vi "get_double_check_moving_by_name.vi"(8 "error in (no error)":errorcluster, 10 "name":string, 11 "MotorSystem in":refnum<class "MotorSystem.lvclass">) -> (0 "error out":errorcluster, 2 "?":cluster{"1st check":bool, "2nd check":bool}, 3 "MotorSystem out":refnum<class "MotorSystem.lvclass">)   [LabVIEW 2016, in "MotionControl.lvlib" / "MotorSystem.lvclass"]
uses:
  <userlib>/MotionControl/MotorSystem/MotorSystem.lvclass
  <userlib>/MotionControl/MotorSystem/MotorSystem.lvclass/MotorSystem.ctl
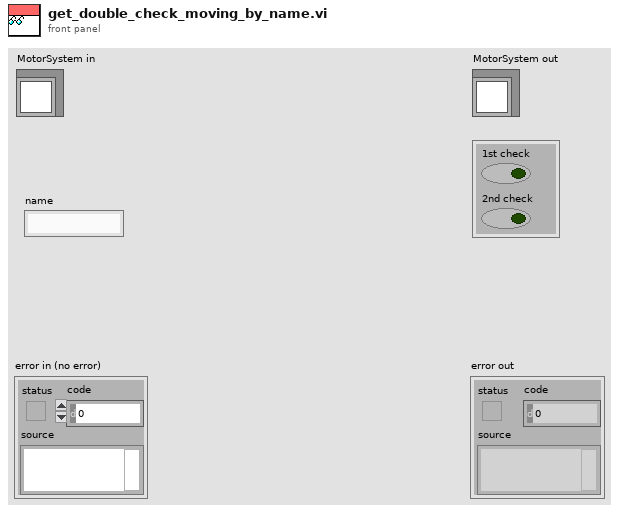
[diagram p1: front panel]
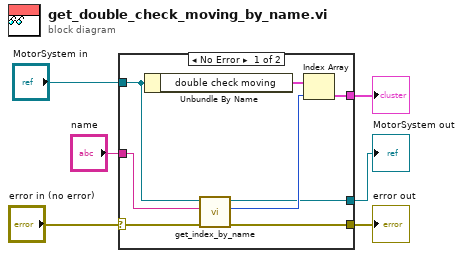
[diagram p0: block diagram]
diagram:
  n1 = case shown="No Error" "error in (no error)" {
    selector: "error in (no error)" -> [w9 w15]
    tunnel: [w8 w15] -> w5
    tunnel: [w7 w16] -> w3
    tunnel: "MotorSystem in" -> [w12 w16]
    tunnel: [w13 _] -> w2
    tunnel: "name" -> [w11 _]
    frame No Error {
      n2 = Unbundle By Name(w12) -> ("double check moving"=w14:cluster{"1st check":bool, "2nd check":bool}[])
      n3 = call <userlib>:"get_index_by_name.vi"("error in (no error)"=w9, "name"=w11, "MotorSystem 输入"=w12) -> ("error out"=w8:errorcluster, "index (0-based)"=w10:u32, "MotorSystem 输出"=w7:refnum<class "MotorSystem.lvclass">)  [unwired: 6 in]
      n4 = Index Array(array=w14, index=w10) -> (element=w13:cluster{"1st check":bool, "2nd check":bool})
    }
    frame Error {
    }
  }
  "error out" <- w5
  "MotorSystem out" <- w3
  "?" <- w2
